vi "OAT RPM Range to Indices.vi"(9 "RPM range in":T2 {"Increment" format="%.2f"; "Maximum" format="%.2f"; "Minimum" format="%.2f"}, 10 "pulse/revolution (1)":dbl=1.0 format="%.2f", 11 "speed profile":T1 {"speed [RPM]" format="%.2f"; "time [s]" format="%.2f"}) -> (1 "RPM scale":cluster{"offset":dbl, "multiplier":dbl} {"multiplier" format="%.2f"; "offset" format="%.2f"}, 2 "rev indices":dbl[](array[numeric]) format="%.2f", 3 "time indices":dbl[](array[numeric]) format="%.2f")   [LabVIEW 2017]
uses:
  <vilib>/addons/Sound and Vibration/Order Analysis/Tach Process/SubVIs/speed profile.ctl
  <vilib>/addons/Sound and Vibration/Order Analysis/Tach Process/SoundVib_TachProcess.lvlib
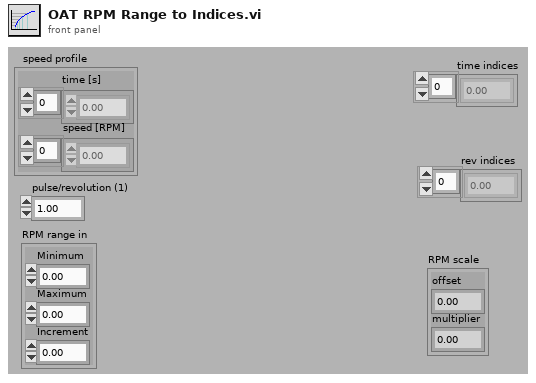
[diagram p1: front panel]
types:
  T1 = typedef "SoundVib_TachProcess.lvlib/speed profile.ctl" = cluster{"time [s]":dbl[], "speed [RPM]":dbl[]}
  T2 = cluster{"Minimum":dbl, "Maximum":dbl, "Increment":dbl}
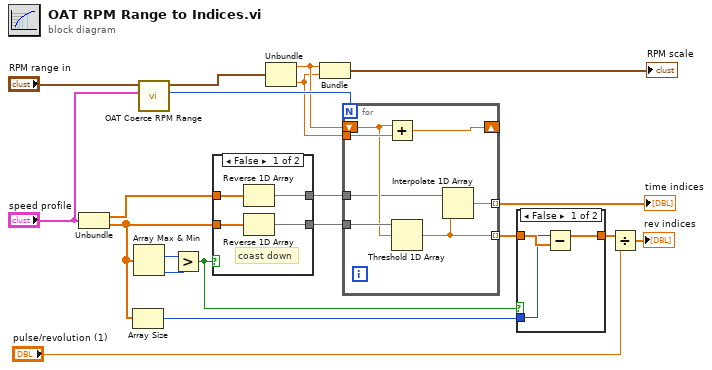
[diagram p0: block diagram]
diagram:
  n1 = Unbundle("speed profile") -> ("time [s]"=w15:dbl[], "speed [RPM]"=w5:dbl[])
  n2 = Array Size(array=w5) -> (size(s)=w1:i32)
  n3 = Array Max & Min(array=w5) -> (max index (indices)=w18:i32, min index (indices)=w17:i32)  [unwired: 2 out]
  n4 = call <vilib>:"OAT Coerce RPM Range.vi"("speed profile"="speed profile", "RPM range in"="RPM range in") -> ("total rpm"=w19:i32, "RPM range out"=w10:T2)  [unwired: 3 in, 1 out]
  n5 = Greater?(x=w18, y=w17) -> (0:w4:bool)
  n6 = case shown="False" w4 {
    tunnel: w5 -> [w23 w26]
    tunnel: [w24 w26] -> w16
    tunnel: w15 -> [w22 w25]
    tunnel: [w21 w25] -> w14
    frame False {
      # "coast down"
      n7 = Reverse 1D Array(array=w22) -> (reversed array=w21:dbl[])
      n8 = Reverse 1D Array(array=w23) -> (reversed array=w24:dbl[])
    }
    frame True {
      # "run up"
    }
  }
  n9 = Unbundle(w10) -> ("Minimum"=w9:dbl, "Increment"=w7:dbl)  [unwired: 1 out]
  n10 = Bundle("Minimum"=w9, "Increment"=w7) -> (→"RPM scale":cluster{"Minimum":dbl, "Increment":dbl})  [unwired: 1 in]
  n11 = for {
    N: w19 -> [_]
    shift-right: [w30] -> _
    shift-left: w9 -> [w31]
    tunnel: w7 -> [w33]
    tunnel: w16 -> [w32]
    tunnel: [w29] -> w3 mode=indexing
    tunnel: w14 -> [w28]
    tunnel: [w27] -> w13 mode=indexing
    n12 = Add(x=w31, y=w33) -> (x+y=w30:dbl)
    n13 = Threshold 1D Array(2:w31, 3:w32) -> (0:w29:dbl)  [unwired: 1 in]
    n14 = Interpolate 1D Array(1:w29, 2:w28) -> (0:w27:dbl)
  }
  "time indices" <- w13
  n15 = case shown="False" w4 {
    tunnel: w3 -> [w36 w37]
    tunnel: [w34 w37] -> w2
    tunnel: w1 -> [w35 _]
    frame False {
      n16 = Subtract(x=w35, y=w36) -> (x-y=w34:dbl[])
    }
    frame True {
    }
  }
  n17 = Divide(x=w2, y="pulse/revolution (1)") -> (x/y=→"rev indices":dbl[])
